vi "Stop Core.vi"(10 "final error code":i32, 11 "reference in":refnum<class "Actor1_Basic_G4_4.0.0.lvclass">) -> (3 "reference out":refnum<class "Actor1_Basic_G4_4.0.0.lvclass">)   [LabVIEW 2012, in "Actor1_Basic_G4_4.0.0.lvlib" / "Actor1_Basic_G4_4.0.0.lvclass"]
uses:
  <resource>/Framework/Providers/Open_GDS/ClassProviders/ActorFramework/4.0.0/Actor1_Basic_G4_4.0.0/Actor1_Basic_G4_4.0.0_class/Actor1_Basic_G4_4.0.0.lvclass
  <vilib>/ActorFramework/Actor/Actor.lvclass
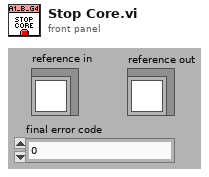
[diagram p1: front panel]
types:
  T1 = typedef "Actor1_Basic_G4_4.0.0.lvlib/Actor1_Basic_G4_4.0.0.lvclass/ObjectAttributes.ctl" = cluster{"None":bool}
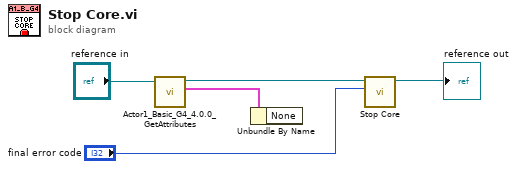
[diagram p0: block diagram]
diagram:
  n1 = call <resource>:"Actor1_Basic_G4_4.0.0_GetAttributes.vi"("reference in"="reference in") -> ("Data"=w4:T1, "reference out"=w3:refnum<class "Actor1_Basic_G4_4.0.0.lvclass">)  [unwired: 7 in, 2 out]
  n2 = Unbundle By Name(w4) -> ()  [unwired: 1 out]
  n3 = call-parent "Stop Core.vi"("final error code"="final error code", "Actor in"=w3) -> ("Actor out"=→"reference out":refnum<class "Actor1_Basic_G4_4.0.0.lvclass">)  [unwired: 9 in]
